vi "GearCollecter_OperatorAssist.vi"(3 "CarriageReturned":bool, 4 "Manual_Overide":bool, 5 "Start":bool, 6 "Gear_Beam_Break_Sensor_Triggered":bool) -> (0 "GearRailCollect":bool, 1 "GearChuteExtend":bool, 2 "Gate_Pos":enum16{"Stop", "Catch", "Clamp", "Open"}(ring))   [LabVIEW 2016]
panel:
  in  "Gear_Collector_State":enum16{"Store Gear", "Wait For Gear", "Idle"}(ring)=enum."Wait For Gear"
  out "Current_State":enum16{"Store Gear", "Wait For Gear", "Idle"}(ring)
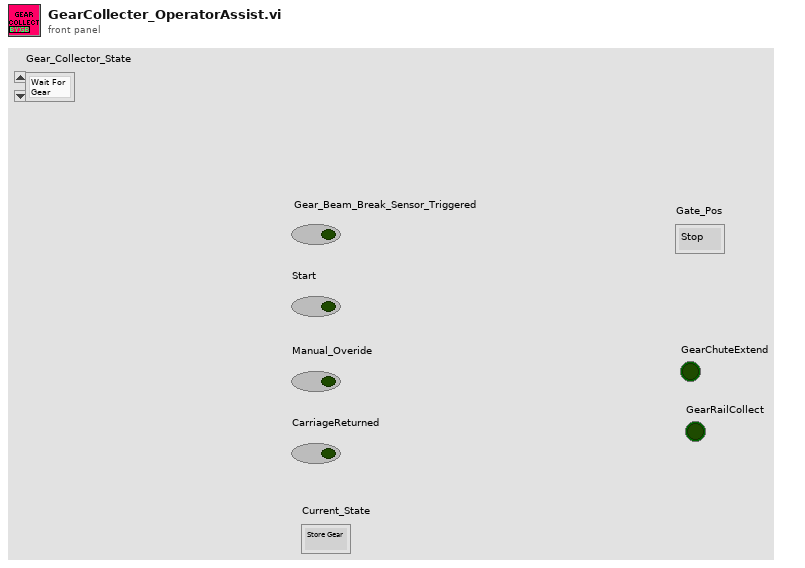
[diagram p1: front panel]
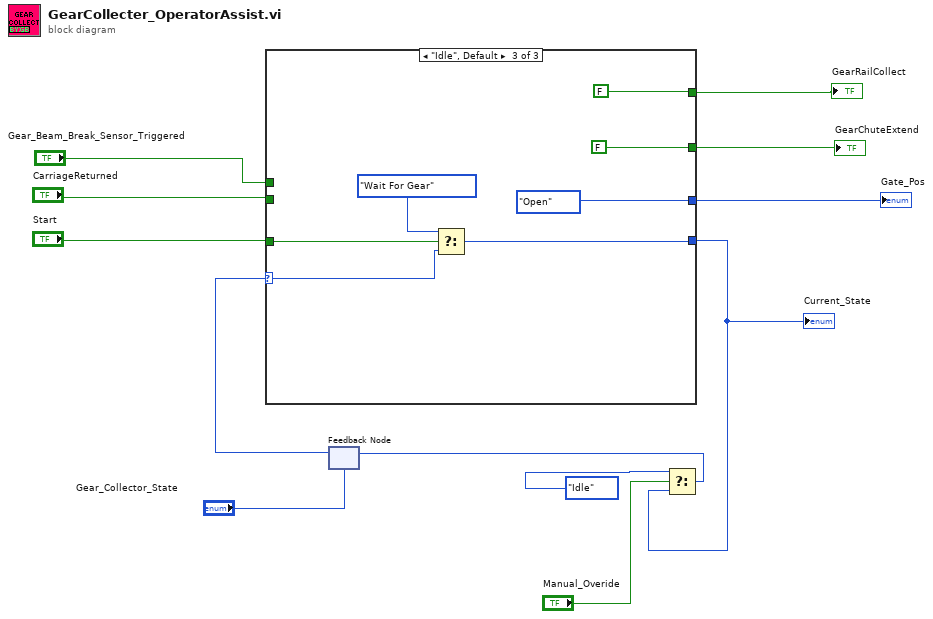
[diagram p0: block diagram]
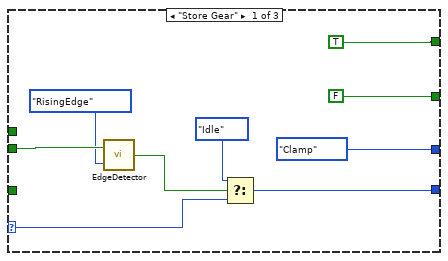
[diagram p2: hidden frame]
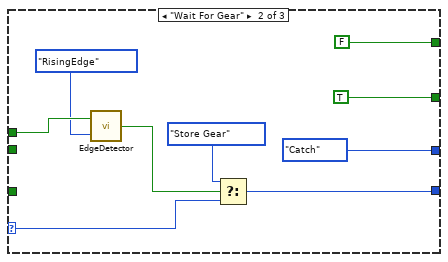
[diagram p3: hidden frame]
diagram:
  n1 = feedback #1("Gear_Collector_State") -> (w11:enum16{"Store Gear", "Wait For Gear", "Idle"})
  n2 = case shown="\"Idle\", Default" w11 {
    selector: w11 -> [w21 w30 w36]
    tunnel: "Start" -> [_ _ w37]
    tunnel: [w19 w28 w34] -> w2
    tunnel: "Gear_Beam_Break_Sensor_Triggered" -> [_ w24 _]
    tunnel: "CarriageReturned" -> [w15 _ _]
    tunnel: [enum16{"Stop", "Catch", "Clamp", "Open"}."Clamp" ("Gate_Pos") enum16{"Stop", "Catch", "Clamp", "Open"}."Catch" ("Gate_Pos") enum16{"Stop", "Catch", "Clamp", "Open"}."Open" ("Gate_Pos")] -> w5
    tunnel: [FALSE ("Extend?") TRUE ("Extend?") FALSE ("Extend?")] -> w4
    tunnel: [TRUE ("Extend?") FALSE ("Extend?") FALSE ("Extend?")] -> w3
    frame "Store Gear" {
      n3 = call "EdgeDetector.vi"("DetectorType"=enum16{"RisingEdge", "FallingEdge", "Both"}."RisingEdge", "Input"=w15) -> ("Edge"=w13:bool)
      n4 = Select(t=enum16{"Store Gear", "Wait For Gear", "Idle"}."Idle", s=w13, f=w21) -> (s? t:f=w19:enum16{"Store Gear", "Wait For Gear", "Idle"})
    }
    frame "Wait For Gear" {
      n5 = call "EdgeDetector.vi"("DetectorType"=enum16{"RisingEdge", "FallingEdge", "Both"}."RisingEdge", "Input"=w24) -> ("Edge"=w22:bool)
      n6 = Select(t=enum16{"Store Gear", "Wait For Gear", "Idle"}."Store Gear", s=w22, f=w30) -> (s? t:f=w28:enum16{"Store Gear", "Wait For Gear", "Idle"})
    }
    frame "Idle", Default {
      n7 = Select(t=enum16{"Store Gear", "Wait For Gear", "Idle"}."Wait For Gear", s=w37, f=w36) -> (s? t:f=w34:enum16{"Store Gear", "Wait For Gear", "Idle"})
    }
  }
  "Gate_Pos" <- w5
  "GearChuteExtend" <- w4
  "GearRailCollect" <- w3
  "Current_State" <- w2
  n8 = Select(t=enum16{"Store Gear", "Wait For Gear", "Idle"}."Idle", s="Manual_Overide", f=w2) -> (s? t:f=w6:enum16{"Store Gear", "Wait For Gear", "Idle"})
  n9 = feedback-in #1(w6) -> ()
